vi "Close MeasurementLink Session.vi"(8 "error in (no error)":errorcluster, 9 "close session behavior":T1, 10 "session in":variant, 11 "instrument in":refnum<class "Instrument.lvclass">) -> (0 "error out":errorcluster)   [LabVIEW 2020, in "MeasurementLink Instrument.lvlib" / "Instrument.lvclass"]
doc: "Closes the local session. If the session represents a remote session, <b>close session behavior</b> determines whether closing the local session closes the server session or detaches from the server session."
uses:
  Instrument.lvclass
  Close Session Behavior.ctl
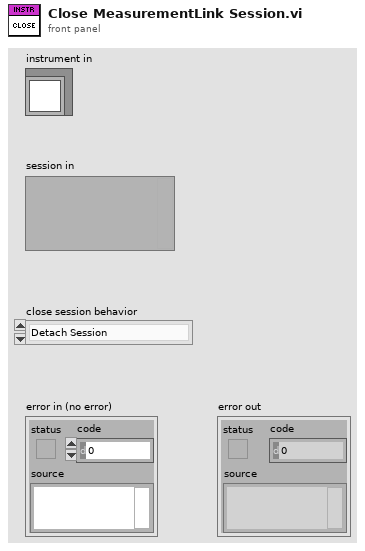
[diagram p1: front panel]
types:
  T1 = typedef "MeasurementLink Instrument.lvlib/Instrument.lvclass/Close Session Behavior.ctl" = enum16{"Detach Session", "Close Session"}
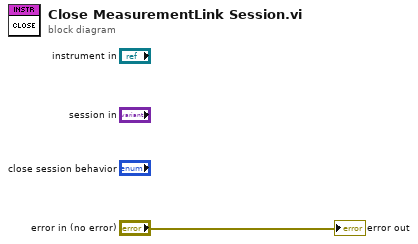
[diagram p0: block diagram]
diagram:
  "error out" <- "error in (no error)"
